vi "DB_ActualizaTablaEquipos.vi"(8 "error in":errorcluster, 11 "Equipos":string[][](array[string])) -> (0 "error out":errorcluster)   [LabVIEW 2018]
uses:
  <vilib>/addons/database/Connection.llb/DB Tools Open Connec (Path).vi
  <vilib>/addons/database/Connection.llb/Conn Execute.vi
  <vilib>/addons/database/Recordset.llb/Rec Destroy - Connection.vi
  <vilib>/addons/database/NI_Database_API.lvlib
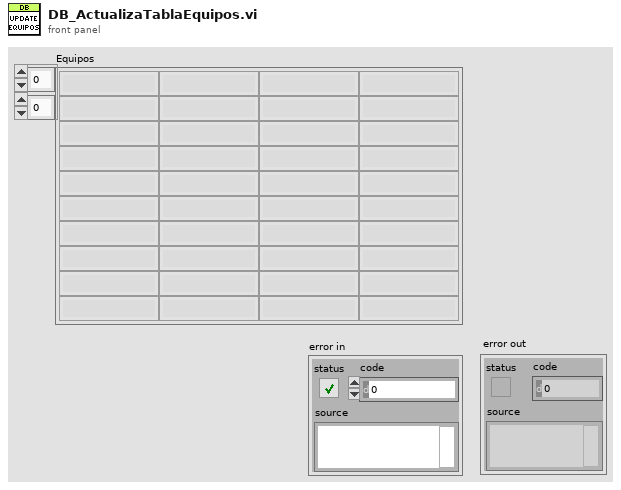
[diagram p1: front panel]
types:
  T1 = typedef "NI_Database_API.lvlib/Conn ObjectReference.ctl" = refnum<k1>
  T2 = typedef "NI_Database_API.lvlib/Rec ObjectReference.ctl" = refnum<k1>
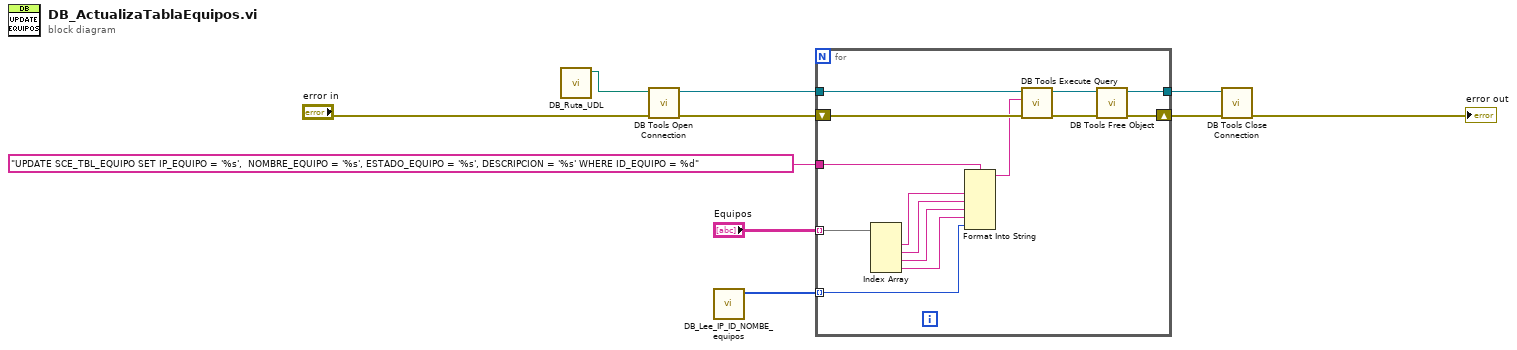
[diagram p0: block diagram]
diagram:
  n1 = call "DB_Ruta_UDL.vi"() -> ("UDL ruta"=w2:path)  [unwired: 11 in]
  n2 = call-poly <vilib>:"DB Tools Open Connection.vi"("error in (no error)"="error in", "connection information"=w2) -> ("error out"=w8:errorcluster, "connection reference"=w6:T1)  [unwired: 6 in]
  n3 = call "DB_Lee_IP_ID_NOMBE_equipos.vi"() -> ("ID_EQUIPO"=w3:i32[])  [unwired: 8 in, 3 out]
  n4 = for {
    tunnel: w6 -> [w22]
    shift-right: [w23] -> w7
    shift-left: w8 -> [w24]
    tunnel: "UPDATE SCE_TBL_EQUIPO SET IP_EQUIPO = '%s',  NOMBRE_EQUIPO = '%s', ESTADO_EQUIPO = '%s', DESCRIPCION = '%s' WHERE ID_EQUIPO = %d" ("SQL") -> [w19]
    tunnel: "Equipos" -> [w17] mode=indexing
    tunnel: w3 -> [w12] mode=indexing
    tunnel: [w11] -> w1
    n5 = Index Array(array=w17) -> (element #1=w13:string, element #2=w16:string, element #3=w15:string, element #4=w14:string)  [unwired: 4 in]
    n6 = Format Into String(format string=w19, w13, w16, w15, w14, w12) -> (resulting string=w18:string)  [unwired: 2 in, 1 out]
    n7 = call-poly <vilib>:"DB Tools Execute Query.vi"("error in (no error)"=w24, "SQL query"=w18, "connection reference"=w22) -> ("error out"=w21:errorcluster, "recordset reference"=w20:T2)  [unwired: 5 in]
    n8 = call-poly <vilib>:"DB Tools Free Object.vi"("error in (no error)"=w21, "recordset reference"=w20) -> ("error out"=w23:errorcluster, "connection reference"=w11:T1)  [unwired: 8 in]
  }
  n9 = call <vilib>:"DB Tools Close Connection.vi"("error in (no error)"=w7, "connection reference"=w1) -> ("error out"=→"error out":errorcluster)  [unwired: 5 in]
